vi "Write IConfiguration.vi"(10 "IConfiguration":refnum<class "IConfiguration.lvclass">, 11 "ConfigurationReference in":refnum<class "ConfigurationReference.lvclass">) -> (3 "ConfigurationReference out":refnum<class "ConfigurationReference.lvclass">)   [LabVIEW 2020, in "Configuration.lvlib" / "ConfigurationReference.lvclass"]
uses:
  <vilib>/gpm_packages/@cs/Configuration/Source/ConfigurationReference/ConfigurationReference.lvclass
  <vilib>/gpm_packages/@cs/Configuration/Source/IConfiguration/IConfiguration.lvclass
  <vilib>/gpm_packages/@cs/Configuration/Source/ConfigurationReference/ConfigurationReference.lvclass/ConfigurationReference.ctl
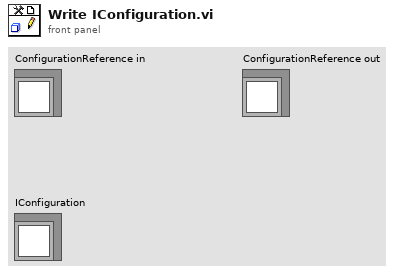
[diagram p1: front panel]
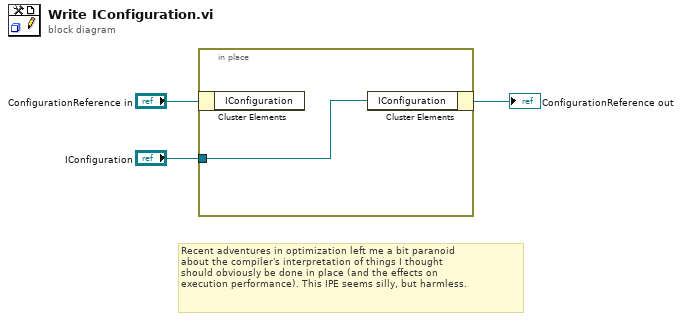
[diagram p0: block diagram]
diagram:
  # "Recent adventures in optimization left me a bit paranoid\nabout the compiler's interpretation of things I thought\nshould obviously be done in place (and the effects on\nexecution performance). This IPE seems silly, but harmless."
  n1 = in-place {
    in-place-border: "IConfiguration" -> [w4]
    n2 = in-place-cluster #1("ConfigurationReference in") -> ()  [unwired: 1 out]
    n3 = in-place-cluster #1("IConfiguration"=w4) -> (→"ConfigurationReference out":refnum<class "ConfigurationReference.lvclass">)
  }
